vi "SVX Polar Plot (N Ch - 1 Order).vi"(0 "magnitudes [RMS]":T9(array[cluster]) {"magnitude" format="%.2f"; "time/rev/RPM" format="%.2f"}, 5 "phases [phase lag]":cluster{"time/rev/RPM":dbl[], "phase":dbl[]}[](array[cluster]) {"phase" format="%.2f"; "time/rev/RPM" format="%.2f"}, 9 "magnitude info":T1[](array[typedef]) {"x-axis units" items=["Time (s)"=0, "Frequency-CB (Hz)"=1, "Frequency-CPB (Hz)"=1248, "Frequency-Arbitrary (Hz)"=2357, "Quefrency (s)"=2, "Revolutions (rev)"=3, "Order"=4, "Speed (RPM)"=11, "Speed (rad/s)"=21, "Index"=65535]; "weighting filter" items=["Linear", "A-weighting", "B-weighting", "C-weighting", "ITU-R 468-4", "Dolby", "CCITT", "C-message", "Wb", "Wc", "Wd", "We", "Wf", "Wh", "Wj", "Wk", "Wm", "AES17 20 kHz lowpass", "AES17 40 kHz lowpass", "AES17 20 kHz highpass", "AES17 40 kHz highpass"]; "dB reference [EU]" format="%.2f"; "engineering units" items=["custom..."=0, "V"=1, "A"=21, "C"=30, "pC"=31, "s"=32, "-"=29, "Pa"=2, "N"=20, "g"=3, "m/s^2"=4, "m/s"=5, "m"=6, "mm/s"=12, "mm"=13, "micron/s"=14, "micron"=15, "in/s^2"=7, "in/s"=8, "in"=9, "mil/s"=10, "mil"=11, "rad/s^2"=16, "rad/s"=17, "rad"=18, "deg/s^2"=26, "deg/s"=27, "deg"=28, "RPM"=22, "cycle/s^2"=23, "Hz"=24, "cycle"=25, "strain"=19]; "spectral info"."window" items=["None "=0, "Hanning"=1, "Hamming"=2, "Blackman-Harris"=3, "Exact Blackman"=4, "Blackman"=5, "Flat Top"=6, "4 Term B-Harris "=7, "7 Term B-Harris"=8, "Low Sidelobe"=9, "Force - Exponential"=10, "Gaussian"=62]}, 11 "error in (no error)":errorcluster, 12 "channel properties":T7[](array[typedef]) {"probe angle [deg]" max=360; "direction" items=["CCW", "CW"]}) -> (3 "unit labels":string[](array[string]), 4 "polar plot":T8(array[cluster]), 15 "error out":errorcluster)   [LabVIEW 2017, in "SoundVib_OAVisualization.lvlib"]
doc: "Prepares polar plot data for displaying on a Polar Plot. Use this VI to show magnitude versus phase for a specific order. Wire data to the <B>magnitudes [RMS]</B> and <B>phases [phase lag]</B> inputs to determine the polymorphic instance to use or manually select the instance."
uses:
  <vilib>/addons/Sound and Vibration/Order Analysis/Data Presentation/SoundVib_OAVisualization.lvlib
  <vilib>/addons/Sound and Vibration/Order Analysis/Data Presentation/SubVIs/OAT MCM Channel Property.ctl
  <vilib>/addons/_NISVFA/_Shared subVIs/Controls/svc_Spectrum Info.ctl
  <vilib>/addons/_NISVFA/_Shared subVIs/Controls/svc_X-Axis Units.ctl
  <vilib>/addons/_NISVFA/_Shared subVIs/Controls/svc_Spectrum Type.ctl
  <vilib>/addons/_NISVFA/_Shared subVIs/Controls/svc_Engineering Units Text Ring.ctl
  <vilib>/addons/_NISVFA/_Shared subVIs/Controls/svc_Weighting Filter Text Ring.ctl
  <vilib>/addons/_NISVFA/_Shared subVIs/Controls/svc_Complimentary Spectrum Units.ctl
  <vilib>/addons/_NISVFA/_Spectrum Processing/SVFA Unit Conversion (XY) (N Ch).vi
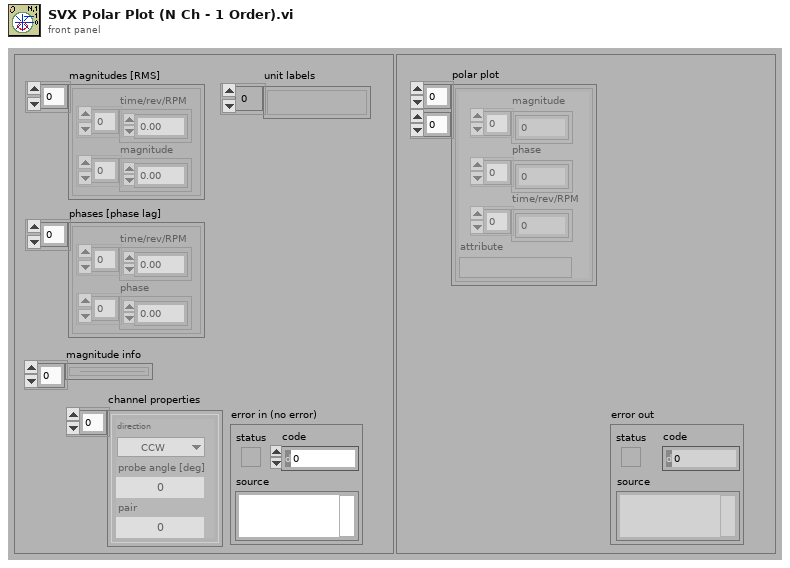
[diagram p1: front panel]
types:
  T1 = typedef "svc_Spectrum Info.ctl" = cluster{"channel name":string, "description":string, "x-axis units":T2, "spectral info":cluster{"spectrum type":T3, "linear/dB":enum16{"linear", "dB"}, "window":u16, "window size":i32, "FFT size":i32}, "engineering units":T4, "custom label":string, "dB reference [EU]":dbl, "peak units":enum16{"rms", "peak", "peak-peak"}, "weighting filter":T5, "spectral density?":bool, "unit label":string, "spectrum skewed?":bool, "complimentary spectrum units":T6}
  T2 = typedef "svc_X-Axis Units.ctl" = u16
  T3 = typedef "svc_Spectrum Type.ctl" = enum16{"FFT Spectrum [complex]", "Amplitude [Magnitude]", "Power [Magnitude^2]", "Cross Spectrum [complex]", "Frequency Response [Complex]"}
  T4 = typedef "svc_Engineering Units Text Ring.ctl" = u16
  T5 = typedef "svc_Weighting Filter Text Ring.ctl" = u16
  T6 = typedef "svc_Complimentary Spectrum Units.ctl" = enum16{"none", "radians", "degrees", "cycles", "imaginary"}
  T7 = typedef "OAT MCM Channel Property.ctl" = cluster{"direction":u16, "probe angle [deg]":u16, "pair":u16}
  T8 = cluster{"magnitude":dbl[], "phase":dbl[], "time/rev/RPM":dbl[], "attribute":variant}[][]
  T9 = cluster{"time/rev/RPM":dbl[], "magnitude":dbl[]}[]
  T10 = cluster{"linear/dB":enum16{"no change", "linear", "dB"}, "dB reference (0: no change)":dbl, "power/magnitude":enum16{"no change", "power", "magnitude"}, "view":enum16{"no change", "rms", "peak", "peak-peak"}}
  T11 = cluster{"magnitude":dbl[], "phase":dbl[], "time/rev/RPM":dbl[], "attribute":variant}
  T12 = cluster{"time/rev/rpm":dbl[], "magnitude":dbl[]}[]
  T13 = cluster{"dB on? (F)":bool, "unwrap phase? (T)":bool, "unit in degree? (T)":bool}
  T14 = cluster{"magnitude":dbl[], "phase":dbl[], "time/rev/RPM":dbl[], "attribute":variant}[]
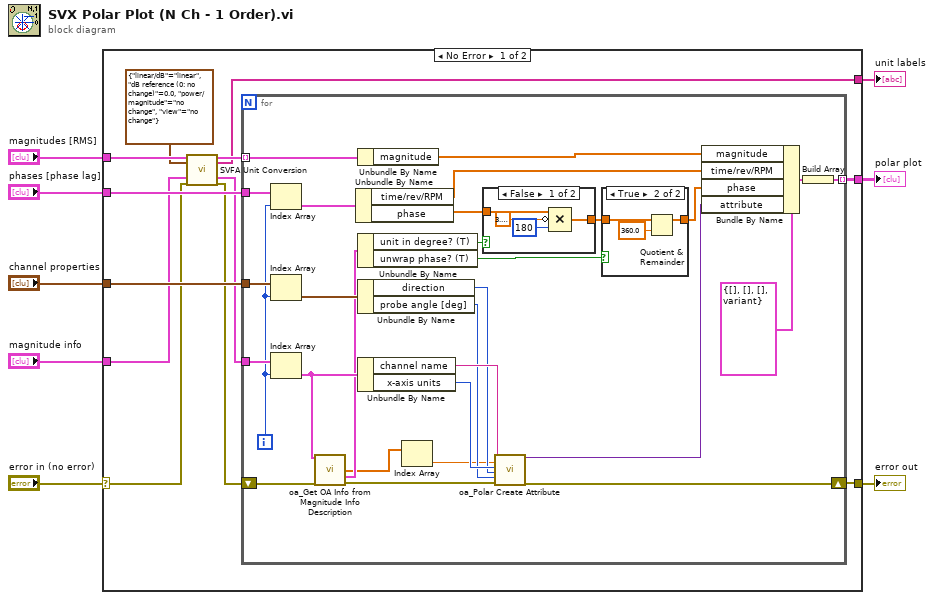
[diagram p0: block diagram]
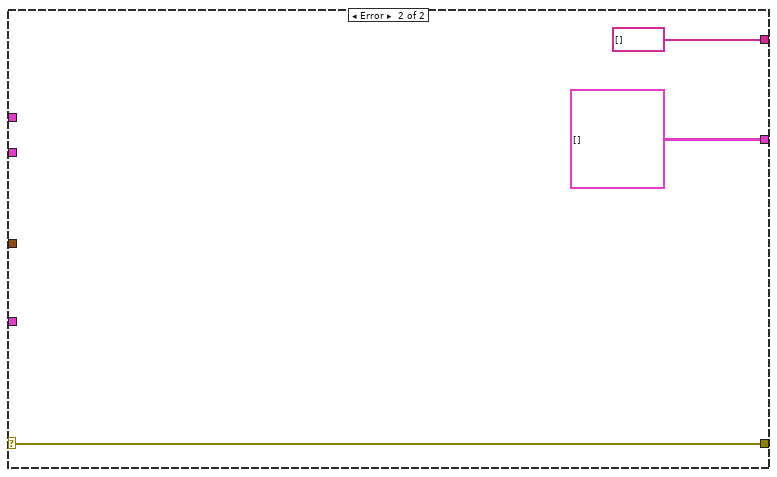
[diagram p4: hidden frame]
diagram:
  n1 = case shown="No Error" "error in (no error)" {
    selector: "error in (no error)" -> [w14 w61]
    tunnel: "magnitudes [RMS]" -> [w16 _]
    tunnel: "phases [phase lag]" -> [w20 _]
    tunnel: "channel properties" -> [w19 _]
    tunnel: [w18 w61] -> w5
    tunnel: [w17 T8 []] -> w2
    tunnel: "magnitude info" -> [w12 _]
    tunnel: [w9 string[] [] ("unit labels")] -> w1
    frame No Error {
      n2 = call-poly <vilib>:"SVFA Unit Conversion.vi"("magnitudes"=w16, "desired scaling"=T10 {"linear/dB"=enum."linear", "dB reference (0: no change)"=0.0, "power/magnitude"=enum."no change", "view"=enum."no change"}, "magnitudes info in"=w12, "error in (no error)"=w14) -> ("converted magnitudes"=w15:T12, "unit labels"=w9:string[], "magnitudes info out"=w11:T1[], "error out"=w13:errorcluster)  [unwired: 12 in]
      n3 = for {
        tunnel: w15 -> [w49] mode=indexing
        tunnel: w20 -> [w45]
        tunnel: w19 -> [w40]
        shift-right: [w31] -> w18
        shift-left: w13 -> [w29]
        tunnel: w11 -> [w43]
        tunnel: [w41] -> w17 mode=indexing
        i -> [w39]
        n4 = Index Array(array=w45, index=w39) -> (element=w44:cluster{"time/rev/RPM":dbl[], "phase":dbl[]})
        n5 = Index Array(array=w40, index=w39) -> (element=w38:T7)
        n6 = Index Array(array=w43, index=w39) -> (element=w27:T1)
        n7 = call <vilib>:"oa_Get OA Info from Magnitude Info Description.vi"("magnitude info"=w27, "error in (no error)"=w29) -> ("orders to compute"=w24:dbl[], "view"=w26:T13, "error out"=w28:errorcluster)  [unwired: 9 in, 2 out]
        n8 = Unbundle By Name(w44) -> ("time/rev/RPM"=w32:dbl[], "phase"=w47:dbl[])
        n9 = Unbundle By Name(w49) -> ("magnitude"=w37:dbl[])
        n10 = Unbundle By Name(w26) -> ("unit in degree? (T)"=w48:bool, "unwrap phase? (T)"=w23:bool)
        n11 = Unbundle By Name(w38) -> ("direction"=w34:u16, "probe angle [deg]"=w33:u16)
        n12 = Unbundle By Name(w27) -> ("channel name"=w36:string, "x-axis units"=w35:T2)
        n13 = Index Array(array=w24) -> (element=w25:dbl)  [unwired: 1 in]
        n14 = case shown="False" w48 {
          tunnel: w47 -> [w57 w58]
          tunnel: [w54 w58] -> w22
          frame False {
            n15 = Compound Arithmetic op=MULTIPLY(w57, invert 3.141592653589793, 180) -> (w54:dbl[])
          }
          frame True {
          }
        }
        n16 = call <vilib>:"oa_Polar Create Attribute.vi"("channel name"=w36, "order"=w25, "x-axis units"=w35, "rotation direction"=w34, "probe angle [deg]"=w33, "error in (no error)"=w28) -> ("attribute out"=w30:variant, "error out"=w31:errorcluster)  [unwired: 12 in]
        n17 = case shown="True" w23 {
          tunnel: [w50 w51] -> w21
          tunnel: w22 -> [w50 w52]
          frame False {
          }
          frame True {
            n18 = Quotient & Remainder(x=w52, y=360.0) -> (x-y*floor(x/y)=w51:dbl[])  [unwired: 1 out]
          }
        }
        n19 = Bundle By Name(cluster=T11 {"magnitude"=[], "phase"=[], "time/rev/RPM"=[], "attribute"=variant} ("element"), "magnitude"=w37, "time/rev/RPM"=w32, "phase"=w21, "attribute"=w30) -> (w42:T11)
        n20 = Build Array(w42) -> (w41:T14)
      }
    }
    frame Error {
    }
  }
  "polar plot" <- w2
  "error out" <- w5
  "unit labels" <- w1
